vi "day 10 task 1.vi"() -> ()   [LabVIEW 2019]
panel:
  out "during":i32[](array[numeric])
  out "Array":i32[](array[numeric])
  out "sum":i32
  out "after":i32[](array[numeric])
  out "tick no.":i32
  out "string array":string[](array[string])
  out "puzzle input":string
  out "size(s)":i32
  # "1,1,4,4,-1"
  # "9-->21\n30-->19"
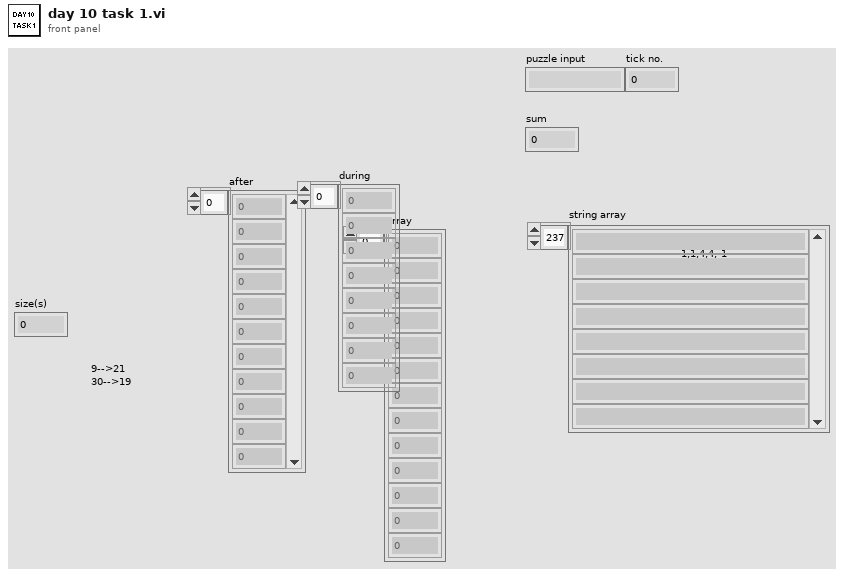
[diagram p1: front panel]
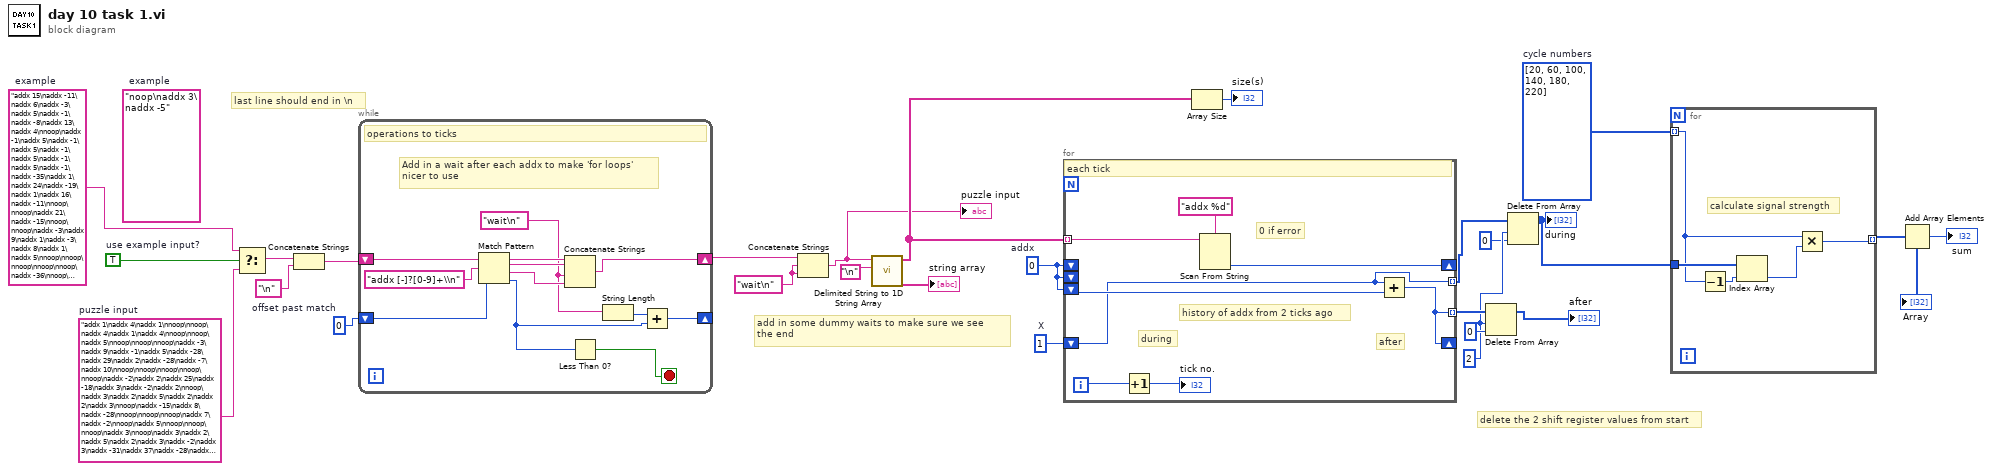
[diagram p0: block diagram]
diagram:
  w8 = i32[] [20, 60, 100, 140, 180, 220]  # cycle numbers
  w4 = 2 ("length")
  w13 = "wait\n" ("regular expression")
  w15 = 1  # X
  w16 = 0  # addx
  w21 = 0  # offset past match
  w1 = "addx 15\naddx -11\naddx 6\naddx -3\naddx 5\naddx -1\naddx -8\naddx 13\naddx 4\nnoop\naddx -1\naddx 5\naddx -1\naddx 5\naddx -1\naddx 5\naddx -1\naddx 5\naddx -1\naddx -35\naddx 1\naddx 24\naddx -19\naddx 1\naddx 16\naddx -11\nnoop\nnoop\naddx 21\naddx -15\nnoop\nnoop\naddx -3\naddx 9\naddx 1\naddx -3\naddx 8\naddx 1\naddx 5\nnoop\nnoop\nnoop\nnoop\nnoop\naddx -36\nnoop\naddx 1\naddx 7\nnoop\nnoop\nnoop\naddx 2\naddx 6\nnoop\nnoop\nnoop\nnoop\nnoop\naddx 1\nnoop\nnoop\naddx 7\naddx 1\nnoop\naddx -13\naddx 13\naddx 7\nnoop\naddx 1\naddx -33\nnoop\nnoop\nnoop\naddx 2\nnoop\nnoop\nnoop\naddx 8\nnoop\naddx -1\naddx 2\naddx 1\nnoop\naddx 17\naddx -9\naddx 1\naddx 1\naddx -3\naddx 11\nnoop\nnoop\naddx 1\nnoop\naddx 1\nnoop\nnoop\naddx -13\naddx -19\naddx 1\naddx 3\naddx 26\naddx -30\naddx 12\naddx -1\naddx 3\naddx 1\nnoop\nnoop\nnoop\naddx -9\naddx 18\naddx 1\naddx 2\nnoop\nnoop\naddx 9\nnoop\nnoop\nnoop\naddx -1\naddx 2\naddx -37\naddx 1\naddx 3\nnoop\naddx 15\naddx -21\naddx 22\naddx -6\naddx 1\nnoop\naddx 2\naddx 1\nnoop\naddx -10\nnoop\nnoop\naddx 20\naddx 1\naddx 2\naddx 2\naddx -6\naddx -11\nnoop\nnoop\nnoop"  # example
  (unwired) "noop\naddx 3\naddx -5"  # example
  w24 = TRUE  # use example input?
  w25 = "addx 1\naddx 4\naddx 1\nnoop\nnoop\naddx 4\naddx 1\naddx 4\nnoop\nnoop\naddx 5\nnoop\nnoop\nnoop\naddx -3\naddx 9\naddx -1\naddx 5\naddx -28\naddx 29\naddx 2\naddx -28\naddx -7\naddx 10\nnoop\nnoop\nnoop\nnoop\nnoop\naddx -2\naddx 2\naddx 25\naddx -18\naddx 3\naddx -2\naddx 2\nnoop\naddx 3\naddx 2\naddx 5\naddx 2\naddx 2\naddx 3\nnoop\naddx -15\naddx 8\naddx -28\nnoop\nnoop\nnoop\naddx 7\naddx -2\nnoop\naddx 5\nnoop\nnoop\nnoop\naddx 3\nnoop\naddx 3\naddx 2\naddx 5\naddx 2\naddx 3\naddx -2\naddx 3\naddx -31\naddx 37\naddx -28\naddx -9\nnoop\nnoop\nnoop\naddx 37\naddx -29\naddx 4\nnoop\naddx -2\nnoop\nnoop\nnoop\naddx 7\nnoop\nnoop\nnoop\naddx 5\nnoop\nnoop\nnoop\naddx 4\naddx 2\naddx 4\naddx 2\naddx 3\naddx -2\nnoop\nnoop\naddx -34\naddx 6\nnoop\nnoop\nnoop\naddx -4\naddx 9\nnoop\naddx 5\nnoop\nnoop\naddx -2\nnoop\naddx 7\nnoop\naddx 2\naddx 15\naddx -14\naddx 5\naddx 2\naddx 2\naddx -32\naddx 33\naddx -31\naddx -2\nnoop\nnoop\naddx 1\naddx 3\naddx 2\nnoop\naddx 2\nnoop\naddx 7\nnoop\naddx 5\naddx -6\naddx 4\naddx 5\naddx 2\naddx -14\naddx 15\naddx 2\nnoop\naddx 3\naddx 4\nnoop\naddx 1\nnoop\nnoop"  # puzzle input
  # "delete the 2 shift register values from start"
  # "add in some dummy waits to make sure we see \nthe end"
  # "last line should end in \\n"
  n1 = Select(t=w1, s=w24, f=w25) -> (s? t:f=w20:string)
  n2 = Concatenate Strings(w20, "\n" ("regular expression")) -> (w18:string)
  n3 = while {
    shift-right: [w34] -> w14
    shift-left: w18 -> [w35]
    shift-right: [w30] -> _
    shift-left: w21 -> [w29]
    stop <- w36 stop-if-true
    w26 = "wait\n" ("regular expression")
    # "Add in a wait after each addx to make 'for loops'\nnicer to use"
    # "operations to ticks"
    n4 = Match Pattern(string=w35, regular expression="addx [-]?[0-9]+\\n", offset (0)=w29) -> (before substring=w33:string, match substring=w28:string, after substring=w32:string, offset past match=w27:i32)
    n5 = Concatenate Strings(w33, w28, w26, w32) -> (w34:string)
    n6 = Less Than 0?(x=w27) -> (x < 0?=w36:bool)
    n7 = String Length(string=w26) -> (length=w31:i32)
    n8 = Add(x=w31, y=w27) -> (x+y=w30:i32)
  }
  n9 = Concatenate Strings(w14, w13, w13) -> (w12:string)
  "puzzle input" <- w12
  n10 = call <vilib>:"Delimited String to 1D String Array.vi"("delimiter"="\n", "delimited string"=w12) -> ("string array"=w17:string[])  [unwired: 9 in]
  "string array" <- w17
  n11 = for {
    tunnel: w17 -> [w45] mode=indexing
    shift-right: [w41] -> _
    shift-left: w16 -> [_]
    shift-left: w16 -> [_]
    shift-left: w16 -> [w40]
    shift-right: [w39] -> _
    shift-left: w15 -> [w38]
    tunnel: [w39] -> w11 mode=indexing
    tunnel: [w38] -> w5 mode=indexing
    i -> [w43]
    # "history of addx from 2 ticks ago"
    # "0 if error"
    # "after"
    # "during"
    # "each tick"
    n12 = Increment(x=w43) -> (x+1=→"tick no.":i32)
    n13 = Scan From String(format string="addx %d", input string=w45) -> (output 1=w41:i32)  [unwired: 3 in, 3 out]
    n14 = Add(x=w38, y=w40) -> (x+y=w39:i32)
  }
  n15 = Array Size(array=w17) -> (size(s)=→"size(s)":i32)
  n16 = Delete From Array(array=w11, length=w4, index=0) -> (array with subset deleted=→"after":i32[])  [unwired: 1 out]
  n17 = Delete From Array(array=w5, length=w4, index=0) -> (array with subset deleted=w2:i32[])  [unwired: 1 out]
  "during" <- w2
  n18 = for {
    tunnel: w2 -> [w50]
    tunnel: w8 -> [w47] mode=indexing
    tunnel: [w46] -> w7 mode=indexing
    # "calculate signal strength"
    n19 = Decrement(x=w47) -> (x-1=w49:i32)
    n20 = Index Array(array=w50, index=w49) -> (element=w48:i32)
    n21 = Multiply(x=w47, y=w48) -> (x*y=w46:i32)
  }
  "Array" <- w7
  n22 = Add Array Elements(numeric array=w7) -> (sum=→"sum":i32)
